vi "_objectTypeStr2Enum.vi"(8 "error in (no error)":errorcluster, 9 "object type":string) -> (0 "error out":errorcluster, 1 "usiObjectType":T1)   [LabVIEW 2020]
uses:
  <vilib>/Platform/storage/utility/usiObjectType.ctl
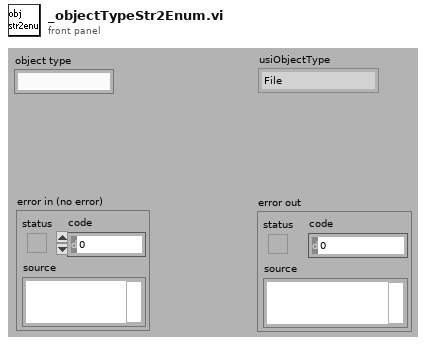
[diagram p1: front panel]
types:
  T1 = typedef "usiObjectType.ctl" = enum16{"File", "Channel Group", "Channel", "Unknown"}
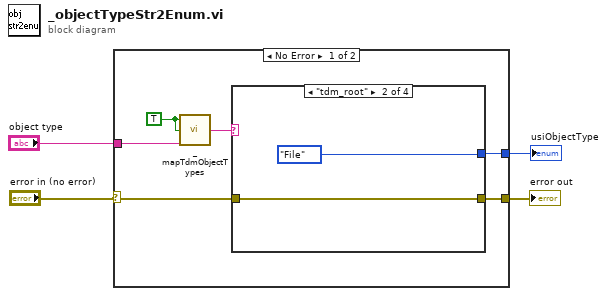
[diagram p0: block diagram]
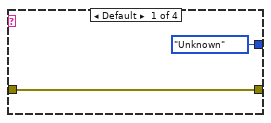
[diagram p2: hidden frame]
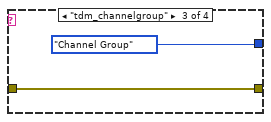
[diagram p3: hidden frame]
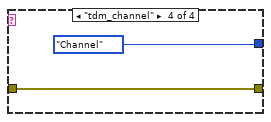
[diagram p4: hidden frame]
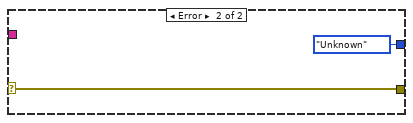
[diagram p5: hidden frame]
diagram:
  n1 = case shown="No Error" "error in (no error)" {
    selector: "error in (no error)" -> [w5 w20]
    tunnel: "object type" -> [w9 _]
    tunnel: [w8 usiObjectType."Unknown" ("usiObjectType")] -> w3
    tunnel: [w7 w20] -> w2
    frame No Error {
      w10 = TRUE ("isTdmDataStructure?")
      n2 = call <vilib>:"_mapTdmObjectTypes.vi"(1:w9, "isTdmDataStructure?"=w10, "DNL_UnMap?(F)"=w10) -> (0:w6:string)
      n3 = case shown="\"tdm_root\"" w6 {
        tunnel: [usiObjectType."Unknown" ("usiObjectType") usiObjectType."File" ("usiObjectType") usiObjectType."Channel Group" ("usiObjectType") usiObjectType."Channel" ("usiObjectType")] -> w8
        tunnel: w5 -> [w11 w13 w15 w17]
        tunnel: [w11 w13 w15 w17] -> w7
        frame Default {
        }
        frame "tdm_root" {
        }
        frame "tdm_channelgroup" {
        }
        frame "tdm_channel" {
        }
      }
    }
    frame Error {
    }
  }
  "usiObjectType" <- w3
  "error out" <- w2
